vi "GT_GetStopDec.vi"(10 "Profile":i16, 11 "rtn_In":cluster{"rtn":i16, "Func":string}) -> (1 "pDecAbruptStop":dbl, 2 "pDecSmoothStop":dbl, 3 "rtn_Out":cluster{"rtn":i16, "Func":string})   [LabVIEW 2014]
uses:
  VC6/gts.dll
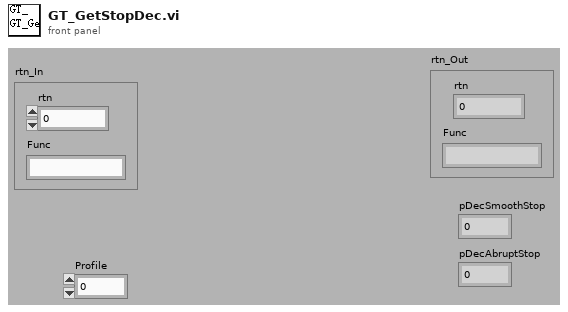
[diagram p1: front panel]
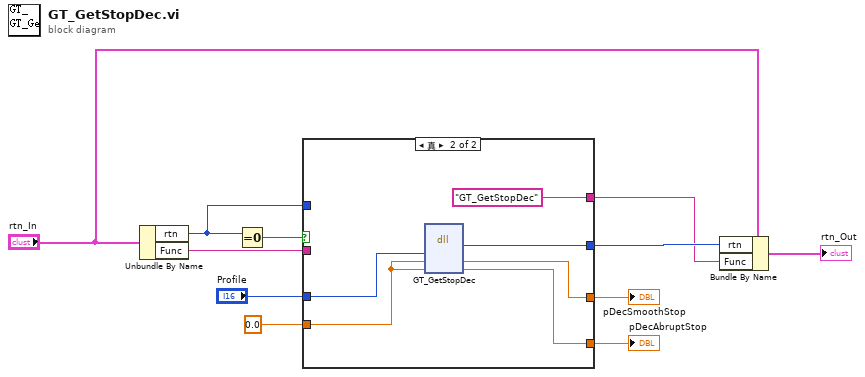
[diagram p0: block diagram]
diagram:
  n1 = Unbundle By Name("rtn_In") -> ("rtn"=w2:i16, "Func"=w10:string)
  n2 = Equal To 0?(x=w2) -> (x = 0?=w11:bool)
  n3 = case shown="真" w11 {
    tunnel: w10 -> [w12 _]
    tunnel: [w13 w20] -> w8
    tunnel: "Profile" -> [_ w19]
    tunnel: [w14 w18] -> w5
    tunnel: [w14 w17] -> w4
    tunnel: 0.0 ("pDecSmoothStop") -> [w14 w16]
    tunnel: w2 -> [w13 _]
    tunnel: [w12 "GT_GetStopDec"] -> w1
    frame False {
    }
    frame True {
      n4 = dll-call lib="PTH2Fabs DNewGTS AC-800LWin7版源程序-20170926gts85VC6gts.dll" fn="GT_GetStopDec"("Profile"=w19, "pDecSmoothStop"=w16, "pDecAbruptStop"=w16) -> ("rtn"=w20:i16, "pDecSmoothStop"=w18:dbl, "pDecAbruptStop"=w17:dbl)  [unwired: 4 in, 2 out]
    }
  }
  "pDecSmoothStop" <- w5
  "pDecAbruptStop" <- w4
  n5 = Bundle By Name(cluster="rtn_In", "rtn"=w8, "Func"=w1) -> (→"rtn_Out":cluster{"rtn":i16, "Func":string})
